vi "log_ratio.vi"(8 "Y":T1 items=["DSRED"=30, "TIME"=0, "FSC"=1, "SSC"=6, "FITC"=9], 9 "X":T1 items=["DSRED"=30, "TIME"=0, "FSC"=1, "SSC"=6, "FITC"=9], 10 "Reactor (INDEX)":i32, 11 "REACTORS":T3) -> (1 "logratio":T2[](array[typedef]), 2 "Median":dbl format="%0.2f", 3 "Updated Reactors":T3)   [LabVIEW 2013]
uses:
  main_machine/type_defs/reactors.ctl
  main_machine/type_defs/reactor.ctl
  main_machine/type_defs/fsc_parameter.ctl
  <vilib>/Analysis/NI_AALBase.lvlib
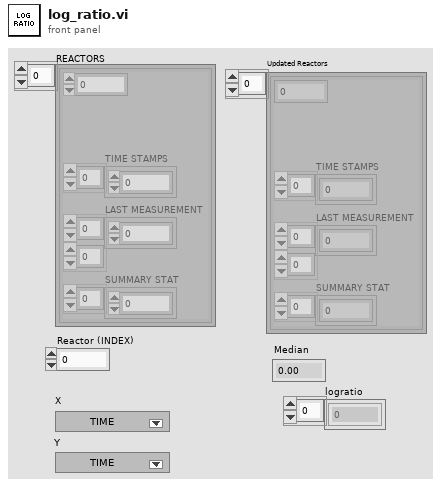
[diagram p1: front panel]
types:
  T1 = typedef "fsc_parameter.ctl" = u16
  T2 = typedef "reactor.ctl" = dbl
  T3 = typedef "reactors.ctl" = cluster{i32, "TIME STAMPS":dbl[], "LAST MEASUREMENT":T2[][], "SUMMARY STAT":dbl[]}[]
  T4 = cluster{i32, "TIME STAMPS":dbl[], "LAST MEASUREMENT":T2[][], "SUMMARY STAT":dbl[]}
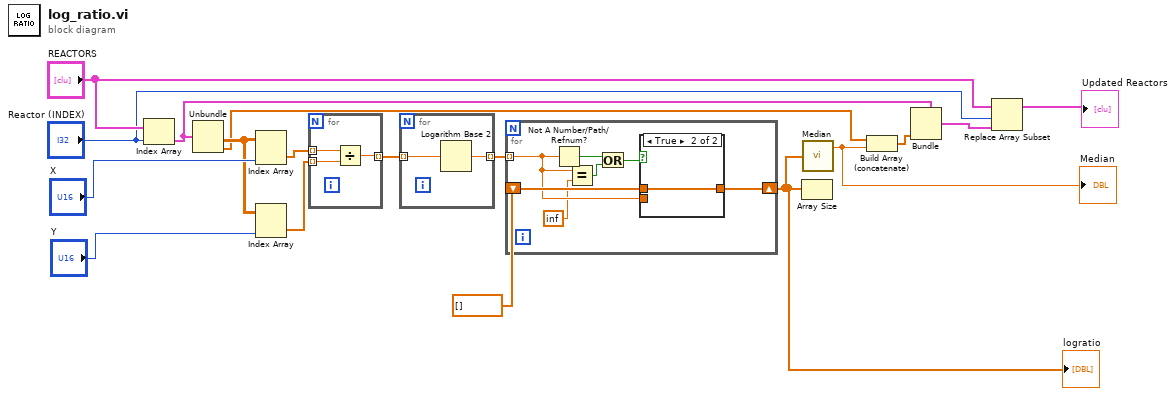
[diagram p0: block diagram]
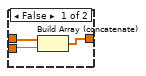
[diagram p2: hidden frame]
diagram:
  n1 = Index Array(array="REACTORS", index="Reactor (INDEX)") -> (element=w17:T4)
  n2 = Unbundle(w17) -> ("LAST MEASUREMENT"=w3:T2[][], "SUMMARY STAT"=w2:dbl[])  [unwired: 2 out]
  n3 = Index Array(array=w3, index (col)="X") -> (element=w16:T2[])  [unwired: 1 in]
  n4 = Index Array(array=w3, index (col)="Y") -> (element=w15:T2[])  [unwired: 1 in]
  n5 = for {
    tunnel: [w20] -> w14 mode=indexing
    tunnel: w15 -> [w19] mode=indexing
    tunnel: w16 -> [w18] mode=indexing
    n6 = Divide(x=w18, y=w19) -> (x/y=w20:T2)
  }
  n7 = for {
    tunnel: w14 -> [w22] mode=indexing
    tunnel: [w21] -> w12 mode=indexing
    n8 = Logarithm Base 2(1:w22) -> (0:w21:T2)
  }
  n9 = for {
    tunnel: w12 -> [w26] mode=indexing
    shift-right: [w28] -> w7
    shift-left: dbl[] [] -> [w29]
    n10 = Not A Number/Path/Refnum?(number/path/refnum=w26) -> (NaN/Path/Refnum?=w27:bool)
    n11 = Equal?(x=w26, y=T2 inf) -> (x = y?=w24:bool)
    n12 = Or(x=w27, y=w24) -> (x .or. y?=w23:bool)
    n13 = case shown="True" w23 {
      tunnel: w29 -> [w32 w33]
      tunnel: [w31 w33] -> w28
      tunnel: w26 -> [w30 _]
      frame False {
        n14 = Build Array (concatenate)(w32, w30) -> (w31:T2[])
      }
      frame True {
      }
    }
  }
  "logratio" <- w7
  n15 = Array Size(array=w7) -> ()  [unwired: 1 out]
  n16 = call <vilib>:"Median.vi"("X"=w7) -> ("median"=w11:dbl)  [unwired: 1 out]
  "Median" <- w11
  n17 = Build Array (concatenate)(w2, w11) -> (w1:dbl[])
  n18 = Bundle(cluster=w17, "SUMMARY STAT"=w1) -> (w13:T4)  [unwired: 3 in]
  n19 = Replace Array Subset(array="REACTORS", new element=w13, index="Reactor (INDEX)") -> (→"Updated Reactors":T3)
